vi "voltmetr_init.vi"(8 "error in (no error)":errorcluster, 11 "UI in":T1) -> (0 "error out":errorcluster, 3 "UI out":T1)   [LabVIEW 2017]
uses:
  ui.ctl
  ui_buttons.ctl
  types/boc_type.ctl
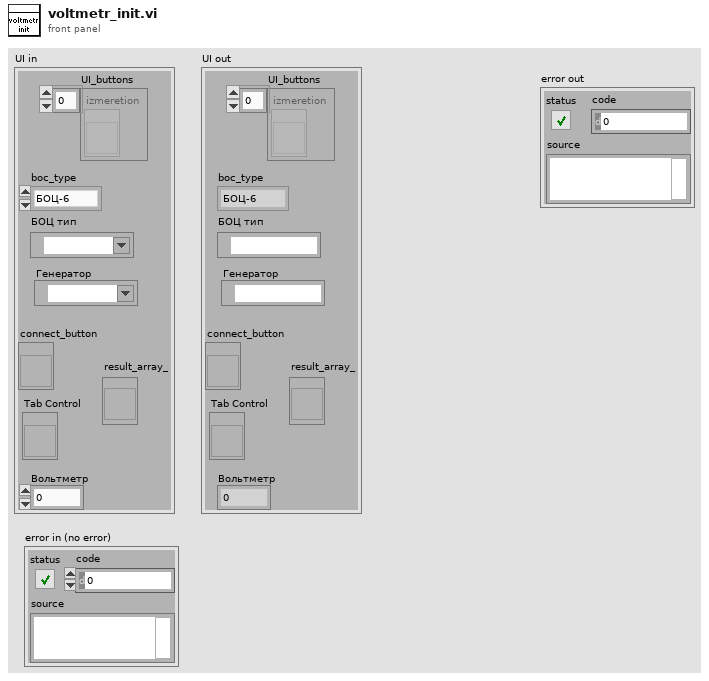
[diagram p1: front panel]
types:
  T1 = typedef "ui.ctl" = cluster{"UI_buttons":T2, "Tab Control":refnum<vi>, "connect_button":refnum<vi>, "generator":refnum<visa-resource-name>, "voltmetr":refnum<visa-resource-name>, "channel_timeout_sec":dbl, "boc_type":T3, "result_array_":refnum<vi>}
  T2 = typedef "ui_buttons.ctl" = refnum<vi>[]
  T3 = typedef "boc_type.ctl" = enum16{"БОЦ-6", "БОЦ-12"}
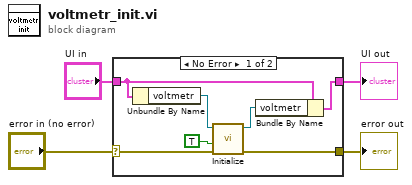
[diagram p0: block diagram]
diagram:
  n1 = case shown="No Error" "error in (no error)" {
    selector: "error in (no error)" -> [w8 w13]
    tunnel: [w11 w12] -> w4
    tunnel: "UI in" -> [w10 w12]
    tunnel: [w6 w13] -> w2
    frame No Error {
      n2 = Unbundle By Name(w10) -> ("voltmetr"=w9:refnum<visa-resource-name>)
      n3 = call <instrlib>:"Initialize.vi"("error in (no error)"=w8, "Reset (True)"=TRUE, "VISA resource name"=w9) -> ("error out"=w6:errorcluster, "VISA resource name out"=w7:refnum<visa-resource-name>)  [unwired: 6 in, 1 out]
      n4 = Bundle By Name(cluster=w10, "voltmetr"=w7) -> (w11:T1)
    }
    frame Error {
    }
  }
  "UI out" <- w4
  "error out" <- w2
